vi "Query Measurement.vi"(8 "error in (no error)":errorcluster, 10 "States":dbl[](array[numeric]), 11 "Agilent E4980 in":refnum<class "Agilent E4980.lvclass">) -> (0 "error out":errorcluster, 1 "Secondary results":dbl[](array[numeric]), 2 "Capacitances (fF)":dbl[](array[numeric]), 3 "Agilent E4980 out":refnum<class "Agilent E4980.lvclass">)   [LabVIEW 2020, in "Agilent E4980.lvclass"]
uses:
  Agilent E4980.lvclass
  C:/Sandbox/Git_Sandbox/WiSpry Test Framework source code (LV20)/WiSpry Test Framework/Instruments/Instrument.lvclass
  Instrument.lvclass/Instrument.ctl
  <instrlib>/Agilent E4980/Agilent E4980.lvlib
  Instrument.lvclass
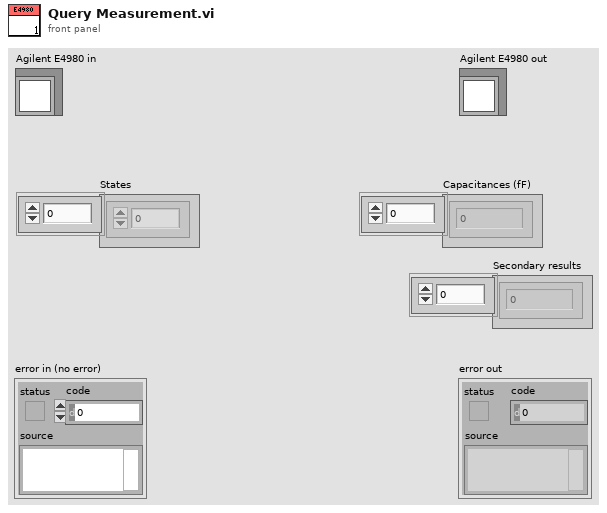
[diagram p1: front panel]
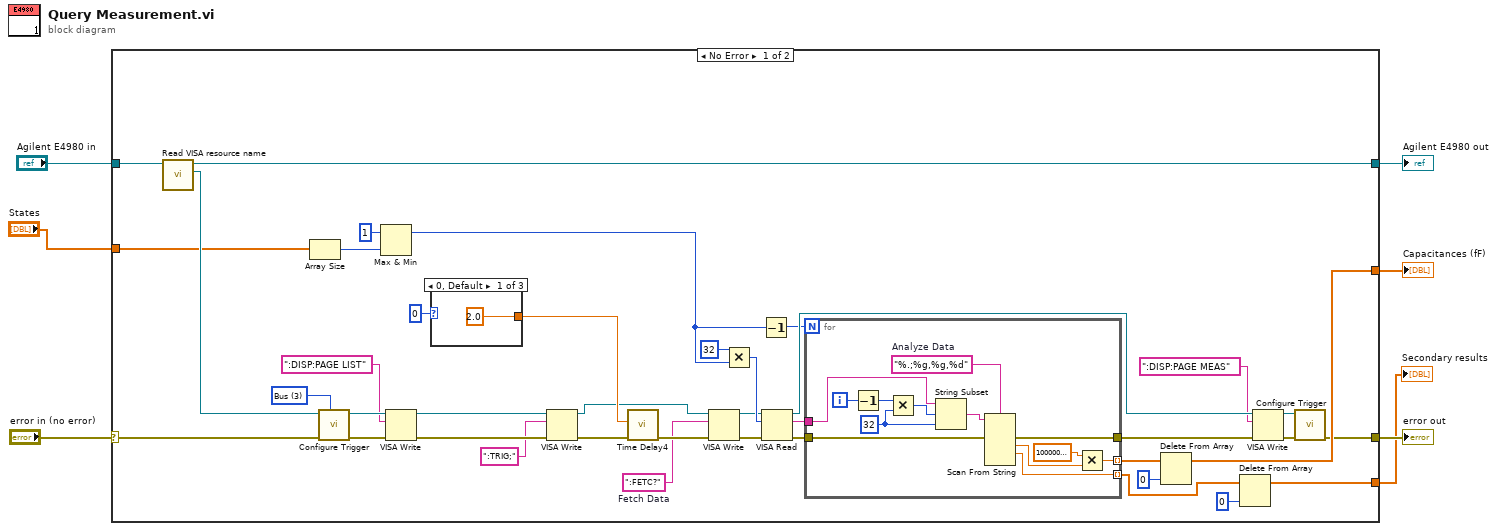
[diagram p0: block diagram]
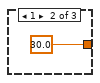
[diagram p2: hidden frame]
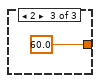
[diagram p3: hidden frame]
diagram:
  n1 = case shown="No Error" "error in (no error)" {
    selector: "error in (no error)" -> [w21 w65]
    tunnel: [w17 w65] -> w6
    tunnel: [w16 w64] -> w5
    tunnel: "Agilent E4980 in" -> [w20 w64]
    tunnel: [w18 _] -> w3
    tunnel: "States" -> [w15 _]
    tunnel: [w11 _] -> w1
    frame No Error {
      w24 = ":FETC?"  # Fetch Data
      w22 = u16 3 items=["Internal", "Manual", "External", "Bus"] ("Trigger Source (0: Internal)")
      n2 = call "Read VISA resource name.vi"("Instrument in"=w20) -> ("VISA resource name"=w19:refnum<visa-resource-name>, "Instrument out"=w16:refnum<class "Agilent E4980.lvclass">)  [unwired: 9 in]
      n3 = Array Size(array=w15) -> (size(s)=w10:i32)
      n4 = call <instrlib>:"Configure Trigger.vi"("Trigger Source (0: Internal)"=w22, "error in (no error)"=w21, "VISA resource name"=w19) -> ("error out"=w29:errorcluster, "VISA resource name out"=w32:refnum<visa-resource-name>)  [unwired: 2 in, 5 out]
      n5 = Max & Min(x=1, y=w10) -> (max(x,y)=w9:i32)  [unwired: 1 out]
      n6 = VISA Write(VISA resource name=w32, write buffer=":DISP:PAGE LIST", error in (no error)=w29) -> (VISA resource name out=w31:refnum<visa-resource-name>, error out=w30:errorcluster)  [unwired: 1 out]
      n7 = case shown="0, Default" u16 0 ("Measurement Time") {
        tunnel: [2.0 ("Delay Time (s)") 30.0 ("Delay Time (s)") 60.0 ("Delay Time (s)")] -> w46
        frame 0, Default {
        }
        frame 1 {
        }
        frame 2 {
        }
      }
      n8 = VISA Write(VISA resource name=w31, write buffer=":TRIG;", error in (no error)=w30) -> (VISA resource name out=w40:refnum<visa-resource-name>, error out=w47:errorcluster)  [unwired: 1 out]
      n9 = call "Time Delay4"("error in (no error)"=w47, "Delay Time (s)"=w46) -> ("error out"=w45:errorcluster)  [unwired: 9 in]
      n10 = VISA Write(VISA resource name=w40, write buffer=w24, error in (no error)=w45) -> (VISA resource name out=w33:refnum<visa-resource-name>, error out=w39:errorcluster)  [unwired: 1 out]
      n11 = Multiply(x=32, y=w9) -> (x*y=w35:i32)
      n12 = Decrement(x=w9) -> (x-1=w38:i32)
      n13 = VISA Read(VISA resource name=w33, byte count=w35, error in (no error)=w39) -> (VISA resource name out=w41:refnum<visa-resource-name>, read buffer=w34:string, error out=w42:errorcluster)  [unwired: 1 out]
      n14 = for {
        N: w38 -> [_]
        tunnel: [w54] -> w44 mode=indexing
        tunnel: w34 -> [w62]
        tunnel: [w56] -> w12 mode=indexing
        tunnel: w42 -> [w52]
        tunnel: [w51] -> w43
        i -> [w58]
        w60 = 32 ("length (rest)")
        w63 = "%.;%g,%g,%d"  # Analyze Data
        n15 = Decrement(x=w58) -> (x-1=w57:i32)
        n16 = Multiply(x=w57, y=w60) -> (x*y=w61:i32)
        n17 = String Subset(string=w62, offset (0)=w61, length (rest)=w60) -> (substring=w59:string)
        n18 = Scan From String(format string=w63, input string=w59, error in=w52) -> (error out=w51:errorcluster, output 1=w55:dbl, output 2=w56:dbl)  [unwired: 1 in, 6 out]
        n19 = Multiply(x=1000000000000000.0, y=w55) -> (x*y=w54:dbl)
      }
      n20 = Delete From Array(array=w44, index=0) -> (array with subset deleted=w18:dbl[])  [unwired: 1 in, 1 out]
      n21 = Delete From Array(array=w12, index=0) -> (array with subset deleted=w11:dbl[])  [unwired: 1 in, 1 out]
      n22 = VISA Write(VISA resource name=w41, write buffer=":DISP:PAGE MEAS", error in (no error)=w43) -> (VISA resource name out=w36:refnum<visa-resource-name>, error out=w37:errorcluster)  [unwired: 1 out]
      n23 = call <instrlib>:"Configure Trigger.vi"("error in (no error)"=w37, "VISA resource name"=w36) -> ("error out"=w17:errorcluster)  [unwired: 3 in, 6 out]
    }
    frame Error {
    }
  }
  "error out" <- w6
  "Agilent E4980 out" <- w5
  "Capacitances (fF)" <- w3
  "Secondary results" <- w1
